vi "Configure Value (Com).vi"(0 "VISA resource name":refnum<visa-resource-name>, 5 "Channel (001)":string="001", 7 "Value At Power On (1: Last Value)":u16(ring)=1 items=["Preset Value", "Last Value"], 9 "Preset Value":dbl min=-9.9999999e+29 max=9.9999999e+29 step=1.0 format="%#_8g", 11 "error in (no error)":errorcluster) -> (4 "VISA resource name out":refnum<visa-resource-name>, 6 "Channel":string, 15 "error out":errorcluster)   [LabVIEW 2020, in "Yokogawa GX Series.lvlib"]
doc: "Sets the preset operation of a communication channel."
uses:
  <instrlib>/Yokogawa GX Series/Yokogawa GX Series.lvlib
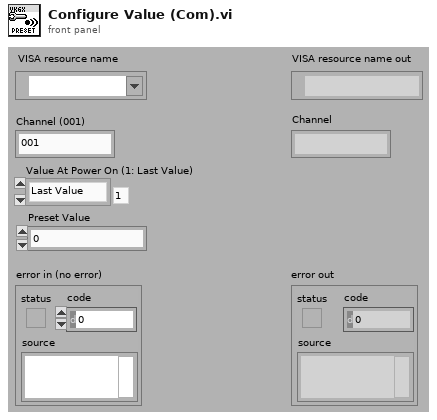
[diagram p1: front panel]
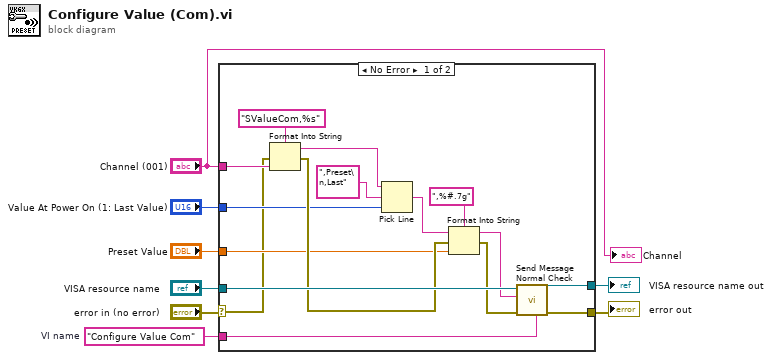
[diagram p0: block diagram]
diagram:
  w7 = "Configure Value Com"  # VI name
  n1 = case shown="No Error" "error in (no error)" {
    selector: "error in (no error)" -> [w9 w25]
    tunnel: "VISA resource name" -> [w24 w26]
    tunnel: w7 -> [w23 _]
    tunnel: [w22 w26] -> w6
    tunnel: [w21 w25] -> w5
    tunnel: "Channel (001)" -> [w12 _]
    tunnel: "Value At Power On (1: Last Value)" -> [w11 _]
    tunnel: "Preset Value" -> [w10 _]
    frame No Error {
      n2 = Format Into String(format string="SValueCom,%s", error in=w9, w12) -> (resulting string=w15:string, error out=w18:errorcluster)  [unwired: 1 in]
      n3 = Pick Line(string ("")=w15, multi-line string=",Preset\n,Last", line index=w11) -> (output string=w13:string)
      n4 = Format Into String(format string=",%#.7g", initial string=w13, error in=w18, w10) -> (resulting string=w17:string, error out=w16:errorcluster)
      n5 = call <instrlib>:"Send Message Normal Check.vi"("Source (\"\")"=w23, "error in (no error)"=w16, "Send Message (\"\")"=w17, "VISA resource name"=w24) -> ("error out"=w21:errorcluster, "VISA resource name out"=w22:refnum<visa-resource-name>)  [unwired: 2 in, 4 out]
    }
    frame Error {
    }
  }
  "error out" <- w5
  "VISA resource name out" <- w6
  "Channel" <- "Channel (001)"
